vi "Generate new url path.vi"(5 "Input Path string":string, 7 "Appending File Path":string, 8 "error in (no error)":errorcluster, 9 "Style/ERD":string, 11 "Refnum":T1) -> (0 "error out":errorcluster, 3 "Ref out":T1)   [LabVIEW 2019]
uses:
  <vilib>/httpClient/ClientHandle.ctl
  <vilib>/regexp/Match Regular Expression.xnode
  <vilib>/httpClient/LabVIEWHTTPClient.lvlib
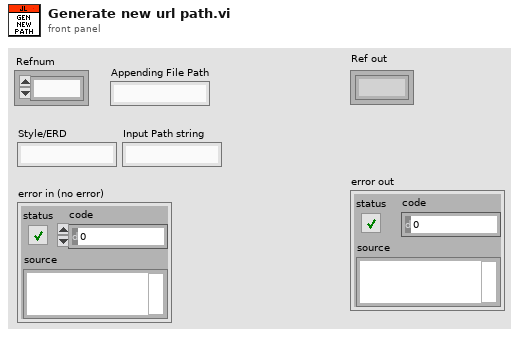
[diagram p1: front panel]
types:
  T1 = typedef "LabVIEWHTTPClient.lvlib/ClientHandle.ctl" = refnum<k1>
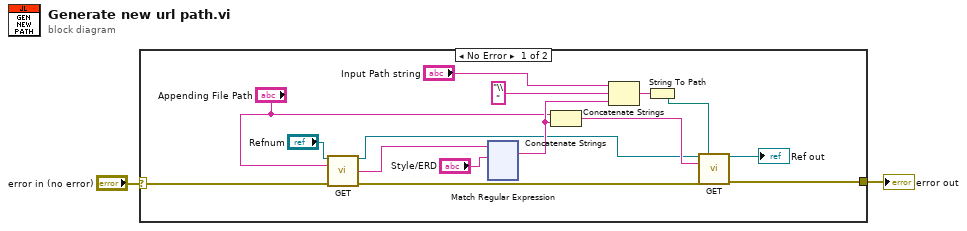
[diagram p0: block diagram]
diagram:
  n1 = case shown="No Error" "error in (no error)" {
    selector: "error in (no error)" -> [w6 w132]
    tunnel: [w5 w132] -> w1
    frame No Error {
      n2 = call <vilib>:"GET.vi"("client handle"="Refnum", "url"="Appending File Path", "error in (no error)"=w6) -> ("client handle out"=w14:T1, "body"=w8:string, "error out"=w12:errorcluster)  [unwired: 9 in, 1 out]
      n3 = xnode "Match Regular Expression"("input string"=w8, "regular expression"="Style/ERD") -> ("whole match"=w15:string)  [unwired: 4 in, 4 out]
      n4 = Concatenate Strings("Appending File Path", w15) -> (w16:string)
      n5 = Concatenate Strings("Input Path string", "\\" ("string"), w15) -> (w11:string)
      n6 = String To Path(string=w11) -> (path=w13:path)
      n7 = call <vilib>:"GET.vi"("client handle"=w14, "output file"=w13, "url"=w16, "error in (no error)"=w12) -> ("client handle out"=→"Ref out":T1, "error out"=w5:errorcluster)  [unwired: 8 in, 2 out]
    }
    frame Error {
    }
  }
  "error out" <- w1
